vi "程序初始化.vi"(11 "端口":u16=3000) -> (1 "数据传输队列":refnum<queue>, 2 "停止位队列":refnum<queue>, 3 "UDP网络连接输出":refnum<k16>, 4 "error out 2":errorcluster caption="错误输出", 5 "初始化数组":i32[][](array[numeric]))   [LabVIEW 2020]
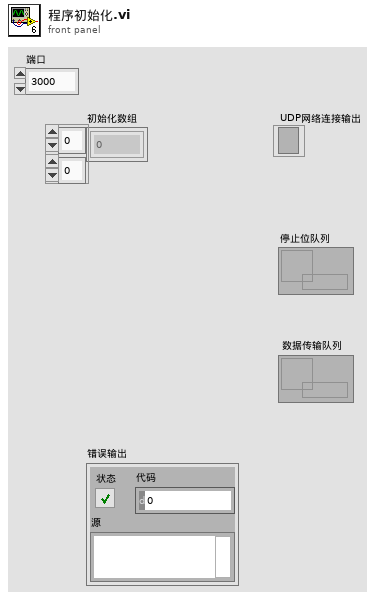
[diagram p1: front panel]
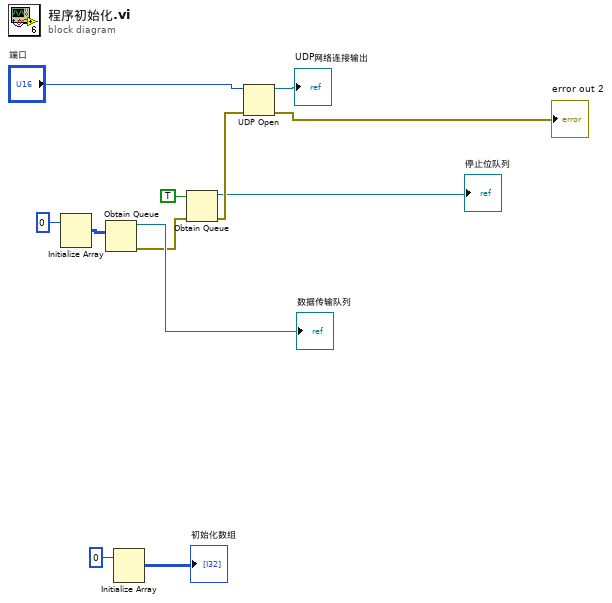
[diagram p0: block diagram]
diagram:
  n1 = Initialize Array(0) -> (w2:i32[][])  [unwired: 2 in]
  n2 = Obtain Queue(element data type=w2) -> (queue out=→"数据传输队列":refnum<queue>, error out=w7:errorcluster)  [unwired: 4 in, 1 out]
  n3 = Initialize Array(0) -> (→"初始化数组":i32[][])  [unwired: 2 in]
  n4 = Obtain Queue(element data type=TRUE, error in (no error)=w7) -> (queue out=→"停止位队列":refnum<queue>, error out=w12:errorcluster)  [unwired: 3 in, 1 out]
  n5 = UDP Open(8:w12, 11:"端口") -> (port=→"UDP网络连接输出":refnum<k16>, 0:→"error out 2":errorcluster)  [unwired: 3 in, 1 out]
